vi "cno_isisubopt.vi"(0 "P":dbl[](array[numeric]), 1 "cno data":T5, 3 "tuning parameters":T1={"constraint weight"=1.0, "maximum minor iterations"=10}, 5 "L":dbl[](array[numeric]), 7 "H":dbl[][](array[numeric]), 9 "OB":dbl[](array[numeric]), 11 "error in (no error)":errorcluster, 12 "PB":dbl[][](array[numeric]), 14 "user defined functions":T2) -> (4 "P":dbl[](array[numeric]), 6 "L":dbl[](array[numeric]), 8 "H":dbl[][](array[numeric]), 10 "number of function calls":i32, 15 "error out":errorcluster)   [LabVIEW 2017, in "NI_Gmath.lvlib"]
uses:
  NI_Gmath.lvlib
  cno_data.ctl
  cno_user defined functions.ctl
  cno_user objective function ref.ctl
  objective function data.ctl
  cno_tuning parameters.ctl
  fpuIEEE64_finiteDiffConstants.ctl
  Real Outer Product.vi
  Real Cholesky Factorization.vi
  A x Vector.vi
  Real A x B.vi
  Full Cholesky Factorization.vi
  Full Real Matrix Cholesky Factorization.vi
  Create Special Real Matrix.vi
  Matrix To Array - RM.vi
  Real Inverse Matrix.vi
  Matrix left divisionMV.vi
  NI_AALBase.lvlib
  NI_AALPro.lvlib
  NI_Matrix.lvlib
panel:
  out "B":dbl[](array[numeric])
  out "G":dbl[](array[numeric])
  out "A":dbl[][](array[numeric])
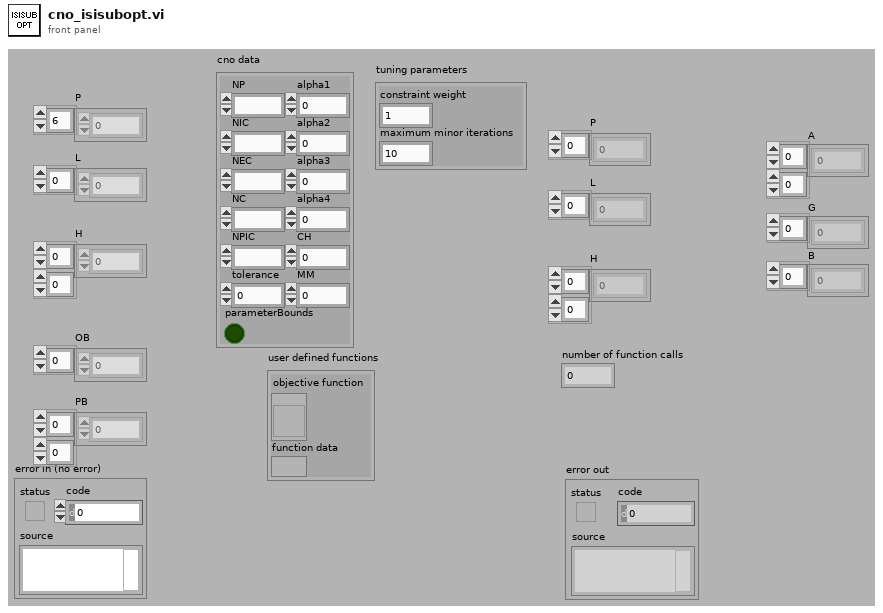
[diagram p1: front panel]
types:
  T1 = typedef "NI_Gmath.lvlib/cno_tuning parameters.ctl" = cluster{"constraint weight":dbl, "maximum minor iterations":i32}
  T2 = typedef "NI_Gmath.lvlib/cno_user defined functions.ctl" = cluster{"objective function":T3, "function data":T4}
  T3 = typedef "NI_Gmath.lvlib/cno_user objective function ref.ctl" = refnum<vi>
  T4 = typedef "NI_Gmath.lvlib/objective function data.ctl" = variant
  T5 = typedef "NI_Gmath.lvlib/cno_data.ctl" = cluster{"NP":i32, "NIC":i32, "NEC":i32, "NC":i32, "NPIC":i32, "parameterBounds":bool, "alpha1":dbl, "alpha2":dbl, "alpha3":dbl, "alpha4":dbl, "CH":i32, "MM":i32, "tolerance":dbl}
  T6 = enum32{"General", "Positive Definite", "Lower Triangular", "Upper Triangular"}
  T7 = enum32{"Identity", "Diagonal", "Toepliz", "Vandermonde", "Companion"}
  T8 = typedef "NI_Gmath.lvlib/fpuIEEE64_finiteDiffConstants.ctl" = dbl
  T9 = typedef "NI_Matrix.lvlib/RealMatrix.ctl" = dbl[][]
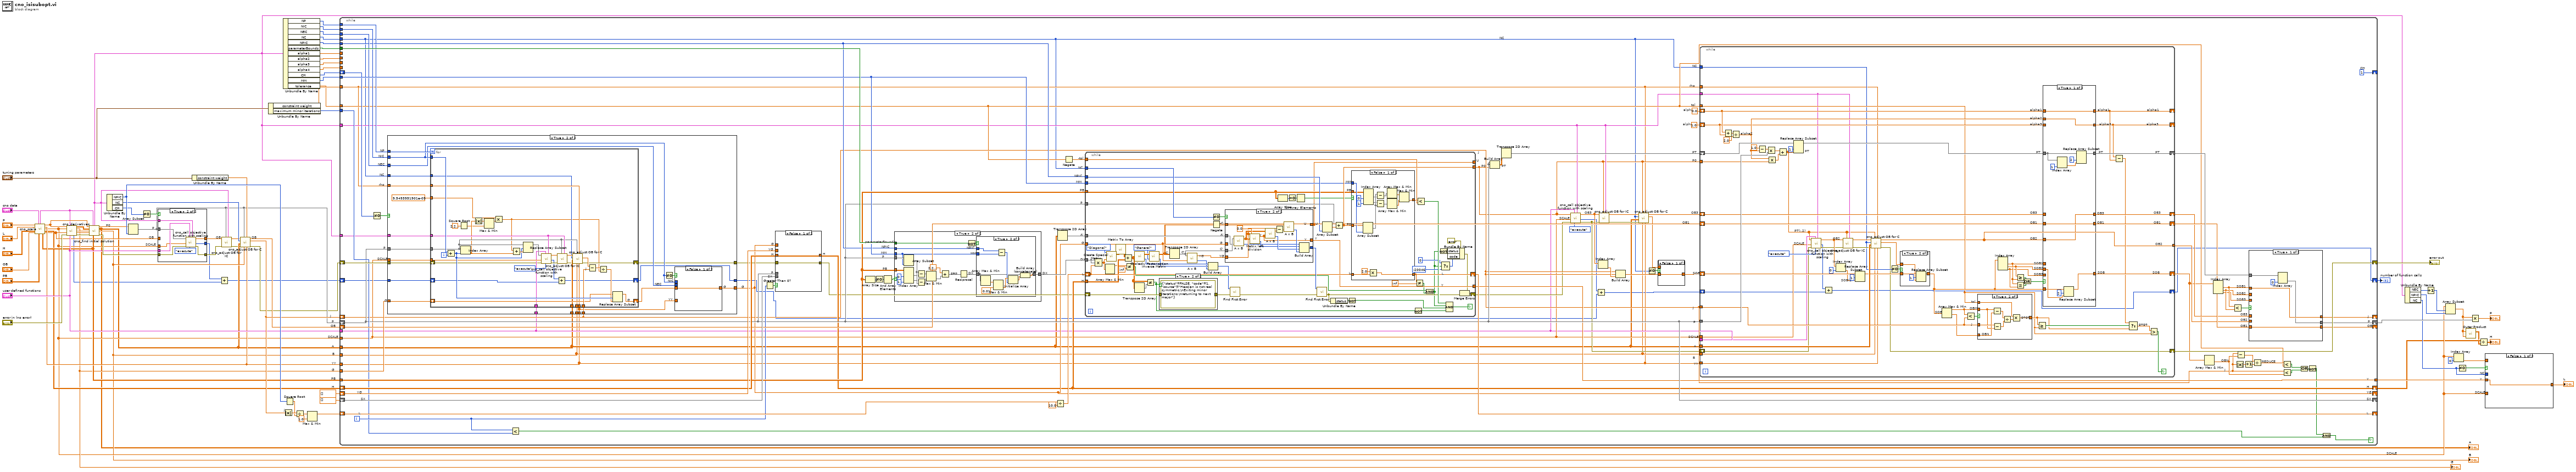
[diagram p0: block diagram]
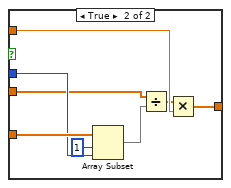
[diagram p2: hidden frame]
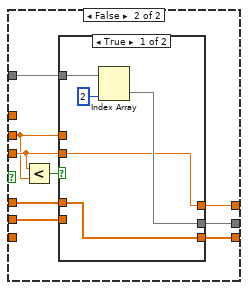
[diagram p3: hidden frame]
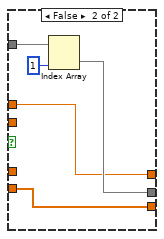
[diagram p4: hidden frame]
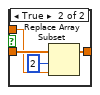
[diagram p5: hidden frame]
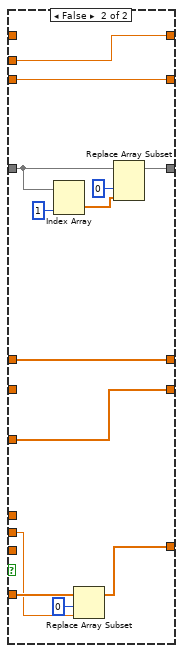
[diagram p6: hidden frame]
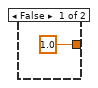
[diagram p7: hidden frame]
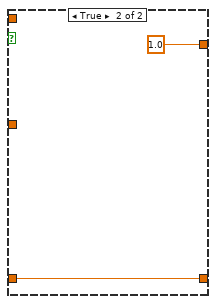
[diagram p9: hidden frame]
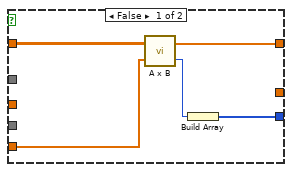
[diagram p10: hidden frame]
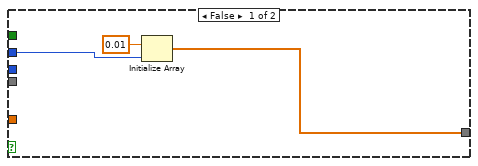
[diagram p12: hidden frame]
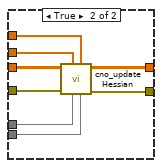
[diagram p14: hidden frame]
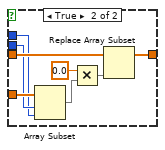
[diagram p16: hidden frame]
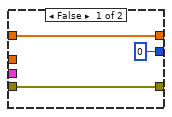
[diagram p17: hidden frame]
diagram:
  # "OB"
  # "NC"
  # "SCALE"
  # "Y"
  # "SCALE"
  # "H"
  # "OB"
  # "OB"
  # "PB"
  # "J"
  # "G"
  # "YY"
  # "B"
  # "A"
  # "SCALE"
  # "P"
  # "J"
  # "P0"
  # "P"
  # "OB"
  # "SCALE"
  n1 = call "cno_scale.vi"("P"="P", "cno data"="cno data", "L"="L", "H"="H", "OB"="OB", "PB"="PB") -> ("cno data"=w66:T5, "P"=w71:dbl[], "L"=w45:dbl[], "SCALE"=w25:dbl[], "H"=w40:dbl[][], "PB"=w43:dbl[][], "OB"=w38:dbl[])  [unwired: 3 in]
  n2 = call "cno_derivatives.vi"("P"=w71, "cno data"=w66, "SCALE"=w25, "OB"=w38, "error in (no error)"="error in (no error)", "user defined functions"="user defined functions") -> ("A"=w70:dbl[][], "G"=w37:dbl[], "B"=w69:dbl[], "CONSTRAINT"=w68:dbl[], "number of function calls"=w3:i32, "error"=w78:errorcluster)  [unwired: 4 in]
  "G" <- w37
  n3 = call "cno_find initial solution.vi"("P0"=w71, "cno data"=w66, "A"=w70, "B"=w69, "CONSTRAINT"=w68, "error"=w78, "PB"=w43) -> ("cno data"=w13:T5, "P0"=w63:dbl[], "A"=w9:dbl[][], "B"=w20:dbl[], "error"=w64:errorcluster)  [unwired: 4 in]
  "A" <- w9
  "B" <- w20
  n4 = Unbundle By Name(w13) -> ("NPIC"=w81:i32, "NC"=w79:i32, "CH"=w14:i32)
  n5 = Array Subset(array=w63, length=w81) -> (w8:dbl[])  [unwired: 1 in]
  n6 = Not Equal To 0?(x=w14) -> (x != 0?=w65:bool)
  n7 = case shown="True" w65 {
    tunnel: w8 -> [_ w93]
    tunnel: w25 -> [_ w90]
    tunnel: "user defined functions" -> [_ w91]
    tunnel: w64 -> [w84 w87]
    tunnel: [w84 w86] -> w10
    tunnel: [w83 w88] -> w12
    tunnel: w38 -> [w83 _]
    tunnel: w13 -> [_ w92]
    tunnel: [0 ("num function calls") w85] -> w4
    frame False {
    }
    frame True {
      n8 = call "cno_call objective function with scaling.vi"("cno data"=w92, "function"=enum16{"initialize", "execute"}."execute", "user defined functions"=w91, "error in (no error)"=w87, "scale"=w90, "X"=w93) -> ("error out"=w86:errorcluster, "num function calls"=w85:i32, "out"=w88:dbl[])  [unwired: 3 in]
    }
  }
  n9 = Unbundle By Name("tuning parameters") -> ("constraint weight"=w44:dbl)
  n10 = Add(x=w4, y=w3) -> (x+y=w2:i32)
  n11 = call "cno_adjust OB for IC.vi"("cno data"=w13, "P"=w8, "error in (no error)"=w10, "OB"=w12) -> ("error out"=w7:errorcluster, "OB"=w11:dbl[])  [unwired: 6 in]
  n12 = call "cno_adjust OB for C.vi"("YY"=w45, "constraint weight"=w44, "B"=w20, "P"=w8, "error in (no error)"=w7, "A"=w9, "NC"=w79, "OB"=w11) -> ("error out"=w6:errorcluster, "J"=w80:dbl, "OB"=w18:dbl[])  [unwired: 1 in]
  n13 = Unbundle By Name("tuning parameters") -> ("constraint weight"=w42:dbl, "maximum minor iterations"=w41:i32)
  n14 = Unbundle By Name(w13) -> ("NP"=w58:i32, "NIC"=w57:i32, "NEC"=w56:i32, "NC"=w54:i32, "NPIC"=w55:i32, "parameterBounds"=w53:bool, "alpha1"=w52:dbl, "alpha2"=w51:dbl, "alpha3"=w50:dbl, "alpha4"=w49:dbl, "CH"=w17:i32, "MM"=w48:i32, "tolerance"=w5:dbl)
  n15 = Absolute Value(x=w80) -> (abs(x)=w61:dbl)
  n16 = Square Root(x=w81) -> (sqrt(x)=w60:dbl)
  n17 = Divide(x=w61, y=w60) -> (x/y=w59:dbl)
  n18 = Max & Min(x=w59, y=1.0) -> (max(x,y)=w39:dbl)  [unwired: 1 out]
  n19 = while {
    tunnel: w58 -> [w137]
    tunnel: w57 -> [w157]
    tunnel: w56 -> [w156]
    tunnel: w55 -> [w155]
    tunnel: w54 -> [w101]
    tunnel: w53 -> [w174]
    tunnel: w52 -> [_]
    tunnel: w51 -> [_]
    tunnel: w50 -> [_]
    tunnel: w49 -> [_]
    tunnel: w48 -> [w167]
    tunnel: "user defined functions" -> [w112]
    tunnel: w25 -> [w113]
    tunnel: w9 -> [w105]
    tunnel: w20 -> [w104]
    tunnel: w45 -> [w103]
    tunnel: w37 -> [w183]
    shift-right: [w185] -> w19
    shift-left: w6 -> [w181]
    shift-right: [w147] -> _
    shift-left: dbl[] [] ("G") -> [w180]
    shift-right: [w148] -> _
    shift-left: dbl[] [] -> [w179]
    shift-right: [w146] -> w23
    shift-left: w40 -> [w178]
    shift-right: [w158] -> _
    shift-left: w39 -> [w173]
    tunnel: w43 -> [w168]
    tunnel: w5 -> [w125]
    shift-right: [w143] -> w33
    shift-left: w8 -> [w148]
    shift-right: [w141] -> _
    shift-left: w18 -> [w159]
    tunnel: w42 -> [w102]
    tunnel: w41 -> [w153]
    shift-right: [w145] -> _
    shift-left: w80 -> [w130]
    tunnel: [w138] -> w30
    shift-right: [1 ("CH")] -> _
    shift-left: w17 -> [w132]
    tunnel: w13 -> [w118]
    tunnel: w13 -> [w110]
    shift-right: [w94] -> w1
    shift-left: w2 -> [w98]
    i -> [w154]
    stop <- w119 continue-if-true
    # "OB"
    # "P"
    # "REDUCE"
    # "J"
    # "OBN"
    # "CH"
    # "J"
    # "Y"
    # "OB3"
    # "OB2"
    # "OB1"
    # "H"
    # "SOB3"
    # "SOB2"
    # "SOB1"
    # "tol"
    # "PT"
    # "J"
    # "rho"
    # "YY"
    # "B"
    # "A"
    # "P0"
    # "NC"
    # "G"
    # "L"
    # "alpha3"
    # "alpha1"
    # "OB3"
    # "SOB"
    # "P"
    # "SCALE"
    # "NC"
    # "OB1"
    # "OB3"
    # "SCALE"
    # "PT"
    # "J"
    # "P0"
    # "U"
    # "DX"
    # "-tol"
    # "MM"
    # "PB"
    # "NPIC"
    # "P"
    # "A'"
    # "NC"
    # "G"
    # "L"
    # "DX"
    # "parameterBounds"
    # "NPIC"
    # "MM"
    # "P"
    # "PB"
    # "L"
    # "H"
    # "P"
    # "H"
    # "H"
    # "SX"
    # "YG"
    # "SX"
    # "YG"
    # "SX"
    # "YG"
    # "G"
    # "G"
    # "rho"
    # "NEC"
    # "SCALE"
    # "P"
    # "NP"
    # "NIC"
    # "NC"
    n20 = Not Equal To 0?(x=w132) -> (x != 0?=w184:bool)
    n21 = case shown="True" w184 {
      tunnel: w137 -> [_ w487]
      tunnel: w148 -> [_ w486]
      tunnel: w157 -> [_ w475]
      tunnel: w112 -> [_ w485]
      tunnel: w113 -> [_ w484]
      tunnel: w101 -> [_ w483]
      tunnel: w156 -> [_ w473]
      tunnel: w105 -> [_ w482]
      tunnel: w104 -> [_ w481]
      tunnel: w103 -> [_ w474]
      tunnel: w102 -> [_ w480]
      tunnel: w130 -> [_ w479]
      tunnel: w183 -> [w465 w478]
      tunnel: [w465 w472] -> w147
      tunnel: w181 -> [w464 w471]
      tunnel: [w464 w470] -> w117
      tunnel: w118 -> [_ w469]
      tunnel: w98 -> [w463 w467]
      tunnel: [w463 w466] -> w96
      frame False {
      }
      frame True {
        w468 = T8 9.5493951901e-09 items=["H_FINITE_DIFF_1"=9.5493951901e-09, "H_FINITE_DIFF_2"=3.2057501263e-06, "H_FINITE_DIFF_4"=0.00033989331283, "H_FINITE_DIFF_K_1"=2.8120287999e-06, "H_FINITE_DIFF_K_2"=9.1341513557e-05, "H_FINITE_DIFF_K_3"=0.00045180790895, "H_FINITE_DIFF_K_4"=0.0014917421406] ("fpuIEEE64")
        # "G"
        # "NIC"
        # "NEC"
        # "YY"
        n22 = for {
          N: w487 -> [_]
          tunnel: w486 -> [w515]
          tunnel: w475 -> [w525]
          tunnel: w485 -> [w521]
          shift-right: [w507] -> w470
          shift-left: w471 -> [w520]
          tunnel: w484 -> [w522]
          tunnel: w483 -> [w514]
          tunnel: w482 -> [w513]
          tunnel: w481 -> [w512]
          tunnel: w474 -> [w511]
          tunnel: w480 -> [w516]
          tunnel: w479 -> [w530]
          shift-right: [w527] -> w476
          shift-left: w478 -> [w526]
          tunnel: w469 -> [w519]
          tunnel: w468 -> [w503]
          shift-right: [w497] -> w466
          shift-left: w467 -> [w498]
          i -> [w533]
          # "G"
          # "J"
          n23 = Add(x=w525, y=w533) -> (x+y=w531:i32)
          n24 = Square Root(x=2.220446049250313e-16) -> (sqrt(x)=w500:dbl)
          n25 = Index Array(array=w515, index=w531) -> (element=w505:dbl)
          n26 = Absolute Value(x=w505) -> (abs(x)=w506:dbl)
          n27 = Max & Min(x=w506, y=w500) -> (max(x,y)=w504:dbl)  [unwired: 1 out]
          n28 = Multiply(x=w503, y=w504) -> (x*y=w502:T8)
          n29 = Add(x=w502, y=w505) -> (x+y=w532:T8)
          n30 = Replace Array Subset(array=w515, new element=w532, index=w531) -> (w524:dbl[])
          n31 = call "cno_call objective function with scaling.vi"("cno data"=w519, "function"=enum16{"initialize", "execute"}."execute", "user defined functions"=w521, "error in (no error)"=w520, "scale"=w522, "X"=w524) -> ("error out"=w508:errorcluster, "num function calls"=w499:i32, "out"=w518:dbl[])  [unwired: 3 in]
          n32 = Add(x=w499, y=w498) -> (x+y=w497:i32)
          n33 = call "cno_adjust OB for IC.vi"("cno data"=w519, "P"=w515, "error in (no error)"=w508, "OB"=w518) -> ("error out"=w509:errorcluster, "OB"=w517:dbl[])  [unwired: 6 in]
          n34 = call "cno_adjust OB for C.vi"("YY"=w511, "constraint weight"=w516, "B"=w512, "P"=w515, "error in (no error)"=w509, "A"=w513, "NC"=w514, "OB"=w517) -> ("error out"=w507:errorcluster, "J"=w510:dbl)  [unwired: 1 in, 1 out]
          n35 = Subtract(x=w510, y=w530) -> (x-y=w529:dbl)
          n36 = Divide(x=w529, y=w502) -> (x/y=w528:T8)
          n37 = Replace Array Subset(array=w526, new element=w528, index=w531) -> (w527:dbl[])
        }
        n38 = Not Equal To 0?(x=w475) -> (x != 0?=w477:bool)
        n39 = case shown="False" w477 {
          tunnel: w476 -> [w488 w496]
          tunnel: w475 -> [_ w493]
          tunnel: w474 -> [_ w495]
          tunnel: w473 -> [_ w494]
          tunnel: [w488 w489] -> w472
          frame False {
          }
          frame True {
            n40 = Array Subset(array=w495, index=w494, length=w493) -> (w492:dbl[])
            n41 = Multiply(x=0.0, y=w492) -> (x*y=w490:dbl[])
            n42 = Replace Array Subset(array=w496, new element=w490) -> (w489:dbl[])  [unwired: 1 in]
          }
        }
      }
    }
    n43 = Less?(x=w154, y=w153) -> (x < y?=w120:bool)
    n44 = Greater Than 0?(x=w154) -> (x > 0?=w182:bool)
    n45 = case shown="False" w182 {
      tunnel: w180 -> [_ w457]
      tunnel: w179 -> [_ w459]
      tunnel: w147 -> [_ w458]
      tunnel: w178 -> [w454 w462]
      tunnel: [w454 w461] -> w146
      tunnel: w148 -> [_ w460]
      tunnel: w117 -> [w453 w456]
      tunnel: [w453 w455] -> w116
      frame False {
      }
      frame True {
        n46 = call "cno_update Hessian.vi"("SX"=w459, "G"=w458, "P"=w460, "YG"=w457, "error in (no error)"=w456, "H"=w462) -> ("error out"=w455:errorcluster, "H"=w461:dbl[][])  [unwired: 4 in]
      }
    }
    n47 = Array Size(array=w168) -> (size(s)=w177:i32[])
    n48 = Not Equal To 0?(x=w177) -> (x != 0?=w176:bool[])
    n49 = And Array Elements(Boolean array=w176) -> (logical AND=w175:bool)
    n50 = case shown="True" w175 {
      tunnel: w168 -> [_ w440]
      tunnel: w148 -> [_ w441]
      tunnel: w167 -> [_ w428]
      tunnel: w174 -> [_ w431]
      tunnel: w155 -> [w423 w427]
      tunnel: [w422 w426] -> w171
      frame False {
        n51 = Initialize Array(0.01 ("element"), w423) -> (w422:dbl[])
      }
      frame True {
        # "NPIC"
        # "MM"
        # "DX"
        # "gap"
        n52 = Array Subset(array=w441, length=w428) -> (w442:dbl[])  [unwired: 1 in]
        n53 = Index Array(array=w440, index (col) #1=0 ("disabled index (col)"), index (col) #2=1 ("index (col)")) -> (element #1=w437:dbl[], element #2=w436:dbl[])  [unwired: 2 in]
        n54 = Subtract(x=w442, y=w437) -> (x-y=w435:dbl[])
        n55 = Subtract(x=w436, y=w442) -> (x-y=w434:dbl[])
        n56 = Max & Min(x=w435, y=w434) -> (min(x,y)=w433:dbl[])  [unwired: 1 out]
        n57 = Add(x=2.220446049250313e-16, y=w433) -> (x+y=w432:dbl[])
        n58 = Reciprocal(x=w432) -> (1/x=w429:dbl[])
        n59 = Not(x=w431) -> (.not. x?=w430:bool)
        n60 = case shown="True" w430 {
          tunnel: w429 -> [w443 w446]
          tunnel: w428 -> [_ w448]
          tunnel: w427 -> [_ w449]
          tunnel: [w443 w444] -> w426
          frame False {
          }
          frame True {
            n61 = Array Max & Min(array=w446) -> (min value=w451:dbl)  [unwired: 3 out]
            n62 = Max & Min(x=w451, y=0.01) -> (min(x,y)=w450:dbl)  [unwired: 1 out]
            n63 = Subtract(x=w449, y=w448) -> (x-y=w447:i32)
            n64 = Initialize Array(w450, w447) -> (w445:dbl[])
            n65 = Build Array (concatenate)(w446, w445) -> (w444:dbl[])
          }
        }
      }
    }
    n66 = Divide(x=w173, y=10.0) -> (x/y=w170:dbl)
    n67 = Transpose 2D Array(2D array=w105) -> (transposed array=w169:dbl[][])
    n68 = Negate(x=w125) -> (-x=w166:dbl)
    n69 = while {
      tunnel: w171 -> [w378]
      shift-right: [w328] -> w114
      shift-left: w116 -> [w375]
      tunnel: w147 -> [w380]
      tunnel: w101 -> [w371]
      tunnel: w169 -> [w368]
      tunnel: w148 -> [w362]
      tunnel: w155 -> [w364]
      tunnel: w168 -> [w358]
      tunnel: w167 -> [w357]
      shift-right: [w337] -> w158
      shift-left: w170 -> [w356]
      tunnel: w166 -> [w354]
      tunnel: [w343] -> _
      tunnel: [w379] -> w108
      tunnel: w146 -> [w342]
      tunnel: [w340] -> w138
      stop <- w352 continue-if-true
      # "Y"
      # "Y"
      # "L"
      # "L"
      # "MM"
      # "PB"
      # "P0"
      # "U"
      # "-C"
      # "G"
      # "YG"
      # "A'"
      # "C'"
      # "C'"
      # "YG"
      # "C"
      n70 = Compound Arithmetic op=MULTIPLY(w378, w378, w356) -> (w326:dbl[])
      n71 = Array Max & Min(array=w326) -> (max value=w325:dbl)  [unwired: 3 out]
      n72 = call-poly "Create Special Matrix.vi"("matrix type"=T7."Diagonal", "Input Vector1"=w326) -> ("Special Matrix"=w339:T9)  [unwired: 3 in, 1 out]
      n73 = call-poly "Matrix To Array.vi"("Real Matrix"=w339) -> ("Real 2D Array"=w338:dbl[][])
      n74 = Add(x=w338, y=w342) -> (x+y=w341:dbl[][])
      n75 = Not Equal?(x=w325, y=inf) -> (x != y?=w323:bool)
      n76 = Transpose 2D Array(2D array=w341) -> (transposed array=w376:dbl[][])
      n77 = call-poly "Cholesky Factorization.vi"("A"=w341) -> ("Cholesky"=w373:T9, "error"=w351:i32)
      n78 = Not Equal?(x=w341, y=w376) -> (x != y?=w374:bool)
      n79 = call-poly "Inverse Matrix.vi"("matrix type"=T6."General", "Input Matrix"=w373) -> ("error"=w350:i32, "Inverse Matrix"=w366:T9)
      n80 = case shown="True" w374 {
        tunnel: w375 -> [w420 _]
        tunnel: [w420 errorcluster {"status"=FALSE, "code"=1, "source"="Hessian is not real symmetric.\nExiting minor iterations,\nreturning to next major"}] -> w347
        frame False {
        }
        frame True {
        }
      }
      n81 = Transpose 2D Array(2D array=w366) -> (transposed array=w369:T9)
      n82 = call-poly "A x B.vi"("Vector"=w380, "A"=w369) -> ("error"=w349:i32, "A x Vector"=w367:dbl[])
      n83 = Build Array(w351, w350, w349) -> (w348:i32[])
      n84 = Not Equal To 0?(x=w371) -> (x != 0?=w370:bool)
      n85 = Negate(x=w366) -> (-x=w365:T9)
      n86 = case shown="True" w370 {
        tunnel: w369 -> [_ w418]
        tunnel: w368 -> [_ w417]
        tunnel: w367 -> [w403 w415]
        tunnel: w380 -> [_ _]
        tunnel: w365 -> [w404 w413]
        tunnel: [w402 w411] -> w343
        tunnel: [w400 w410] -> w381
        tunnel: [_ w405] -> w340
        frame False {
          n87 = call-poly "A x B.vi"("Vector"=w403, "A"=w404) -> ("error"=w401:i32, "A x Vector"=w402:dbl[])
          n88 = Build Array(w401) -> (w400:i32[])
        }
        frame True {
          # "Y"
          # "U"
          # "Y"
          n89 = call-poly "A x B.vi"("B"=w417, "A"=w418) -> ("error"=w406:i32, "A x B"=w416:T9)
          n90 = call-poly "Matrix left division.vi"("A"=w415, "B"=w416, "SVD relative tolerance"=0.0) -> ("error"=w407:i32, "B\\A"=w405:dbl[])  [unwired: 1 in]
          n91 = call-poly "A x B.vi"("Vector"=w405, "A"=w416) -> ("error"=w408:i32, "A x Vector"=w414:dbl[])
          n92 = Subtract(x=w415, y=w414) -> (x-y=w412:dbl[])
          n93 = call-poly "A x B.vi"("Vector"=w412, "A"=w413) -> ("error"=w409:i32, "A x Vector"=w411:dbl[])
          n94 = Build Array(w406, w407, w408, w409) -> (w410:i32[])
        }
      }
      n95 = call "Find First Error.vi"("error in (no error)"=w347, "error codes"=w348) -> ("error out"=w346:errorcluster)  [unwired: 2 in, 1 out]
      n96 = Array Size(array=w358) -> (size(s)=w361:i32[])
      n97 = Equal To 0?(x=w361) -> (x = 0?=w360:bool[])
      n98 = Or Array Elements(Boolean array=w360) -> (logical OR=w359:bool)
      n99 = call "Find First Error.vi"("error in (no error)"=w346, "error codes"=w381) -> ("error out"=w329:errorcluster)  [unwired: 2 in, 1 out]
      n100 = Array Subset(array=w343, length=w364) -> (w363:dbl[])  [unwired: 1 in]
      n101 = Unbundle By Name(w329) -> ("status"=w345:bool)
      n102 = Add(x=w362, y=w363) -> (x+y=w379:dbl[])
      n103 = Not(x=w345) -> (.not. x?=w344:bool)
      n104 = case shown="False" w359 {
        tunnel: w379 -> [w393 _]
        tunnel: w358 -> [w394 _]
        tunnel: w357 -> [w396 _]
        tunnel: w356 -> [w391 w399]
        tunnel: [w389 w399] -> w337
        tunnel: [w384 1.0] -> w355
        frame False {
          n105 = Array Subset(array=w393, length=w396) -> (w397:dbl[])  [unwired: 1 in]
          n106 = Index Array(array=w394, index (col) #1=0 ("disabled index (col)"), index (col) #2=1 ("index (col)")) -> (element #1=w383:dbl[], element #2=w382:dbl[])  [unwired: 2 in]
          n107 = Multiply(x=2.0, y=w391) -> (x*y=w389:dbl)
          n108 = Subtract(x=w397, y=w383) -> (x-y=w387:dbl[])
          n109 = Subtract(x=w382, y=w397) -> (x-y=w388:dbl[])
          n110 = Array Max & Min(array=w387) -> (min value=w386:dbl)  [unwired: 3 out]
          n111 = Array Max & Min(array=w388) -> (min value=w385:dbl)  [unwired: 3 out]
          n112 = Max & Min(x=w386, y=w385) -> (min(x,y)=w384:dbl)  [unwired: 1 out]
        }
        frame True {
        }
      }
      n113 = Not(x=w374) -> (.not. x?=w353:bool)
      n114 = Not Equal?(x=w337, y=inf) -> (x != y?=w321:bool)
      n115 = Less?(x=w355, y=w354) -> (x < y?=w335:bool)
      n116 = And(x=w323, y=w321) -> (x .and. y?=w322:bool)
      n117 = Not(x=w322) -> (.not. x?=w334:bool)
      n118 = Select(t=0, s=w322, f=-20046 ("t")) -> (s? t:f=w331:i32)
      n119 = Compound Arithmetic op=AND(w335, w322, w344, w353) -> (w352:bool)
      n120 = Bundle By Name(cluster=errorcluster {"status"=FALSE, "code"=0, "source"=""} ("error constant"), "status"=w334, "code"=w331) -> (w327:errorcluster)
      n121 = Merge Errors(w327, w329) -> (w328:errorcluster)
    }
    n122 = Build Array(w148, w148, w108) -> (w165:dbl[][])
    n123 = Transpose 2D Array(2D array=w165) -> (transposed array=w164:dbl[][])
    n124 = call "cno_call objective function with scaling.vi"("cno data"=w110, "function"=enum16{"initialize", "execute"}."execute", "user defined functions"=w112, "error in (no error)"=w114, "scale"=w113, "X"=w108) -> ("error out"=w107:errorcluster, "num function calls"=w97:i32, "out"=w111:dbl[])  [unwired: 3 in]
    n125 = Add(x=w97, y=w96) -> (x+y=w95:i32)
    n126 = Index Array(array=w111) -> (element=w162:dbl)  [unwired: 1 in]
    n127 = call "cno_adjust OB for IC.vi"("cno data"=w110, "P"=w108, "error in (no error)"=w107, "OB"=w111) -> ("error out"=w106:errorcluster, "OB"=w109:dbl[])  [unwired: 6 in]
    n128 = Build Array(w130, w130, w162) -> (w161:dbl[])
    n129 = call "cno_adjust OB for C.vi"("YY"=w103, "constraint weight"=w102, "B"=w104, "P"=w108, "error in (no error)"=w106, "A"=w105, "NC"=w101, "OB"=w109) -> ("J"=w100:dbl, "OB"=w99:dbl[])  [unwired: 1 in, 1 out]
    n130 = Not Equal To 0?(x=w101) -> (x != 0?=w163:bool)
    n131 = case shown="False" w163 {
      tunnel: w161 -> [w210 w214]
      tunnel: [w210 w212] -> w160
      tunnel: w100 -> [_ w211]
      frame False {
      }
      frame True {
        n132 = Replace Array Subset(array=w214, new element=w211, index=2) -> (w212:dbl[])
      }
    }
    n133 = while {
      tunnel: w113 -> [w231]
      tunnel: w148 -> [w275]
      shift-right: [w243] -> w142
      shift-left: w159 -> [w246]
      tunnel: w112 -> [w232]
      tunnel: w101 -> [w226]
      tunnel: w108 -> [w274]
      shift-right: [w245] -> w144
      shift-left: w164 -> [w271]
      shift-right: [w218] -> w185
      shift-left: w107 -> [w233]
      tunnel: w105 -> [w280]
      tunnel: w104 -> [w223]
      tunnel: w103 -> [w222]
      tunnel: w102 -> [w224]
      tunnel: w130 -> [w262]
      shift-right: [w252] -> w134
      shift-left: w160 -> [w268]
      tunnel: w125 -> [w236]
      shift-right: [w244] -> w139
      shift-left: w99 -> [w247]
      shift-right: [w240] -> _
      shift-left: 0.0 -> [w251]
      shift-right: [w241] -> _
      shift-left: 1.0 -> [w249]
      tunnel: [w220] -> w140
      tunnel: w110 -> [w229]
      shift-right: [w215] -> w94
      shift-left: w95 -> [w216]
      stop <- w235 continue-if-true
      # "OB2"
      # "PT(:,2)"
      # "alpha3"
      # "alpha1"
      # "OB3"
      # "PT"
      # "OB1"
      # "gogo"
      # "alpha3"
      # "alpha1"
      # "SOB"
      # "PT"
      # "OB3"
      # "OB1"
      # "OB1"
      # "OB2"
      # "OB3"
      # "PT"
      # "alpha3"
      # "alpha2"
      # "alpha1"
      # "SOB"
      # "SOB3"
      # "SOB2"
      # "SOB1"
      # "tol"
      # "J"
      # "OBM"
      # "SOB"
      # "SOB(1)"
      # "OB2"
      # "PT"
      # "alpha2"
      # "SCALE"
      n134 = Add(x=w251, y=w249) -> (x+y=w279:dbl)
      n135 = Divide(x=w279, y=2.0) -> (x/y=w250:dbl)
      n136 = Subtract(x=1.0, y=w250) -> (x-y=w276:dbl)
      n137 = Multiply(x=w276, y=w275) -> (x*y=w273:dbl[])
      n138 = Multiply(x=w250, y=w274) -> (x*y=w272:dbl[])
      n139 = Add(x=w273, y=w272) -> (x+y=w221:dbl[])
      n140 = Replace Array Subset(array=w271, new element=w221, index (col)=1 ("disabled index (col)")) -> (w248:dbl[][])  [unwired: 1 in]
      n141 = call "cno_call objective function with scaling.vi"("cno data"=w229, "function"=enum16{"initialize", "execute"}."execute", "user defined functions"=w232, "error in (no error)"=w233, "scale"=w231, "X"=w221) -> ("error out"=w225:errorcluster, "num function calls"=w217:i32, "out"=w230:dbl[])  [unwired: 3 in]
      n142 = Add(x=w217, y=w216) -> (x+y=w215:i32)
      n143 = Index Array(array=w230, index=0) -> (element=w266:dbl)
      n144 = call "cno_adjust OB for IC.vi"("cno data"=w229, "P"=w221, "error in (no error)"=w225, "OB"=w230) -> ("error out"=w227:errorcluster, "OB"=w228:dbl[])  [unwired: 6 in]
      n145 = Replace Array Subset(array=w268, new element=w266, index=1) -> (w264:dbl[])
      n146 = call "cno_adjust OB for C.vi"("YY"=w222, "constraint weight"=w224, "B"=w223, "P"=w221, "error in (no error)"=w227, "A"=w280, "NC"=w226, "OB"=w228) -> ("error out"=w218:errorcluster, "J"=w219:dbl, "OB"=w220:dbl[])  [unwired: 1 in]
      n147 = Not Equal To 0?(x=w226) -> (x != 0?=w265:bool)
      n148 = case shown="True" w265 {
        tunnel: w264 -> [w316 w320]
        tunnel: [w316 w318] -> w259
        tunnel: w219 -> [_ w317]
        frame False {
        }
        frame True {
          n149 = Replace Array Subset(array=w320, new element=w317, index=1) -> (w318:dbl[])
        }
      }
      n150 = Array Max & Min(array=w259) -> (max value=w261:dbl, min value=w260:dbl)  [unwired: 2 out]
      n151 = Less?(x=w261, y=w262) -> (x < y?=w263:bool)
      n152 = case shown="True" w263 {
        tunnel: w262 -> [_ w314]
        tunnel: w261 -> [_ w313]
        tunnel: w260 -> [_ w315]
        tunnel: w236 -> [_ w308]
        tunnel: [1.0 w309] -> w239
        frame False {
        }
        frame True {
          # "gogo"
          # "OBN"
          n153 = Subtract(x=w313, y=w315) -> (x-y=w312:dbl)
          n154 = Subtract(x=w314, y=w313) -> (x-y=w311:dbl)
          n155 = Divide(x=w312, y=w311) -> (x/y=w310:dbl)
          n156 = Multiply(x=w308, y=w310) -> (x*y=w309:dbl)
        }
      }
      n157 = Index Array(array=w259) -> (element #1=w257:dbl, element #2=w258:dbl, element #3=w256:dbl)  [unwired: 3 in]
      n158 = Greater Or Equal?(x=w258, y=w257) -> (x >= y?=w255:bool)
      n159 = Less Or Equal?(x=w257, y=w256) -> (x <= y?=w254:bool)
      n160 = Or(x=w255, y=w254) -> (x .or. y?=w253:bool)
      n161 = Greater Or Equal?(x=w239, y=w236) -> (x >= y?=w242:bool)
      n162 = case shown="True" w253 {
        tunnel: w259 -> [w293 w306]
        tunnel: w220 -> [w283 w296]
        tunnel: w257 -> [_ _]
        tunnel: w256 -> [_ _]
        tunnel: w258 -> [w291 w304]
        tunnel: [w290 w303] -> w252
        tunnel: w251 -> [w281 _]
        tunnel: w250 -> [w282 w294]
        tunnel: w249 -> [_ w302]
        tunnel: [w282 w302] -> w241
        tunnel: w248 -> [w288 w300]
        tunnel: [w285 w297] -> w245
        tunnel: w247 -> [_ w295]
        tunnel: w246 -> [w284 _]
        tunnel: [w283 w295] -> w244
        tunnel: [w284 w296] -> w243
        tunnel: [w281 w294] -> w240
        frame True {
          n163 = Index Array(array=w288, index (col)=1 ("disabled index (col)")) -> (element=w286:dbl[])  [unwired: 1 in]
          n164 = Replace Array Subset(array=w293, new element=w291, index=2) -> (w290:dbl[])
          n165 = Replace Array Subset(array=w288, new element=w286, index (col)=2 ("disabled index (col)")) -> (w285:dbl[][])  [unwired: 1 in]
        }
        frame False {
          n166 = Index Array(array=w300, index (col)=1 ("disabled index (col)")) -> (element=w298:dbl[])  [unwired: 1 in]
          n167 = Replace Array Subset(array=w306, new element=w304, index=0) -> (w303:dbl[])
          n168 = Replace Array Subset(array=w300, new element=w298, index (col)=0 ("disabled index (col)")) -> (w297:dbl[][])  [unwired: 1 in]
        }
      }
      n169 = Subtract(x=w241, y=w240) -> (x-y=w238:dbl)
      n170 = Select(t=w238, s=w242, f=w239) -> (s? t:f=w237:dbl)
      n171 = Greater?(x=w237, y=w236) -> (0:w235:bool)
    }
    n172 = Array Max & Min(array=w134) -> (min value=w131:dbl)  [unwired: 3 out]
    n173 = Index Array(array=w134) -> (element #1=w152:dbl, element #2=w151:dbl, element #3=w150:dbl)  [unwired: 3 in]
    n174 = Less?(x=w152, y=w151) -> (x < y?=w149:bool)
    n175 = Absolute Value(x=w130) -> (abs(x)=w129:dbl)
    n176 = Subtract(x=w130, y=w131) -> (x-y=w128:dbl)
    n177 = Increment(x=w129) -> (x+1=w127:dbl)
    n178 = case shown="True" w149 {
      tunnel: w152 -> [w190 _]
      tunnel: w151 -> [_ w192]
      tunnel: w150 -> [_ w196]
      tunnel: [w190 w195] -> w145
      tunnel: w144 -> [w189 w199]
      tunnel: [w188 w198] -> w143
      tunnel: w142 -> [w187 _]
      tunnel: [w187 w194] -> w141
      tunnel: w140 -> [_ w191]
      tunnel: w139 -> [_ w193]
      frame True {
        n179 = Index Array(array=w189, index (col)=0 ("disabled index (col)")) -> (element=w188:dbl[])  [unwired: 1 in]
      }
      frame False {
        n180 = Less?(x=w196, y=w192) -> (x < y?=w197:bool)
        n181 = case shown="True" w197 {
          tunnel: w199 -> [w204 w209]
          tunnel: [w202 w207] -> w198
          tunnel: w196 -> [w201 _]
          tunnel: [w201 w206] -> w195
          tunnel: [w200 w205] -> w194
          tunnel: w193 -> [w200 _]
          tunnel: w192 -> [_ w206]
          tunnel: w191 -> [_ w205]
          frame True {
            n182 = Index Array(array=w204, index (col)=2 ("disabled index (col)")) -> (element=w202:dbl[])  [unwired: 1 in]
          }
          frame False {
            n183 = Index Array(array=w209, index (col)=1 ("disabled index (col)")) -> (element=w207:dbl[])  [unwired: 1 in]
          }
        }
      }
    }
    n184 = Divide(x=w128, y=w127) -> (x/y=w126:dbl)
    n185 = Less?(x=w126, y=w125) -> (x < y?=w124:bool)
    n186 = Less?(x=w130, y=w131) -> (x < y?=w123:bool)
    n187 = Or(x=w124, y=w123) -> (x .or. y?=w122:bool)
    n188 = Not(x=w122) -> (.not. x?=w121:bool)
    n189 = And(x=w121, y=w120) -> (x .and. y?=w119:bool)
  }
  "error out" <- w19
  "number of function calls" <- w1
  n190 = Unbundle By Name(w13) -> ("NEC"=w35:i32, "NPIC"=w36:i32, "NC"=w29:i32)
  n191 = Increment(x=w35) -> (x+1=w34:i32)
  n192 = Array Subset(array=w25, index=w34, length=w36) -> (w27:dbl[])
  n193 = Index Array(array=w25, index=0) -> (element=w24:dbl)
  n194 = Not Equal To 0?(x=w29) -> (x != 0?=w31:bool)
  n195 = call-poly "Outer Product.vi"("Y Vector"=w27, "X Vector"=w27) -> ("Outer Product"=w22:T9)  [unwired: 1 out]
  n196 = Multiply(x=w27, y=w33) -> (x*y=→"P":dbl[])
  n197 = Divide(x=w23, y=w22) -> (x/y=→"H":T9)
  n198 = case shown="False" w31 {
    tunnel: w30 -> [w534 w538]
    tunnel: w25 -> [_ w541]
    tunnel: w29 -> [_ w539]
    tunnel: [w534 w535] -> w28
    tunnel: w24 -> [_ w542]
    frame False {
    }
    frame True {
      n199 = Array Subset(array=w541, index=1, length=w539) -> (w537:dbl[])
      n200 = Divide(x=w538, y=w537) -> (x/y=w536:dbl[])
      n201 = Multiply(x=w536, y=w542) -> (x*y=w535:dbl[])
    }
  }
  "L" <- w28
